vi "Normal Coefficient of Variation PDF SDV.vi"(8 "error in":errorcluster, 10 "n":i32=100, 11 "CV":dbl=0.21) -> (0 "error out":errorcluster={"status"=FALSE, "code"=-23026, "source"="Scale range exceeded"}, 1 "Baseline":dbl, 2 "SDV":dbl, 3 "Mean":dbl, 4 "Fit Result String":string="CV PDF  Gaussian LM Least Square Fit:\nAmplitude: 25.528592 ± 0.013986\nCenter: 0.210423 ± 9.838581E-6\nSDV: 0.015489 ± 9.825245E-6\nFWHM: 0.036473 ± 2.313668E-5\nIntegral: 991.140471\nMSE: 0.060195\nR^2: 0.999786\n")   [LabVIEW 2021, in "Math.lvlib"]
uses:
  Math.lvlib
  85f3da7c-8858-4d9f-a12c-d9901bcd4fde.vi
  Fits/Fits.lvlib
  <vilib>/Utility/miscctls.llb/LVPointDoubleTypeDef.ctl
  Fits/Fit Models.ctl
  Fits/Fit Plot Request Information.ctl
  Arrays/Linear Ramp End Options.ctl
  Arrays/Arrays.lvlib
  Fits/Nonlinear Fit Method.ctl
  Fits/Ramp Type.ctl
  Fits/Residual Type.ctl
  Fits/Non-linear Fitting Algorithm.ctl
  Fits/Fit Settings.ctl
  Fits/IRF(X)PSED/Fit Weights Type v2.ctl
panel:
  out "Fit Parameter Values":dbl[](array[numeric])
  out "XY Graph":cluster{"X Array":dbl[], "Y Array":dbl[]}[](graph)
  in  "# Steps (1)":i32=1000
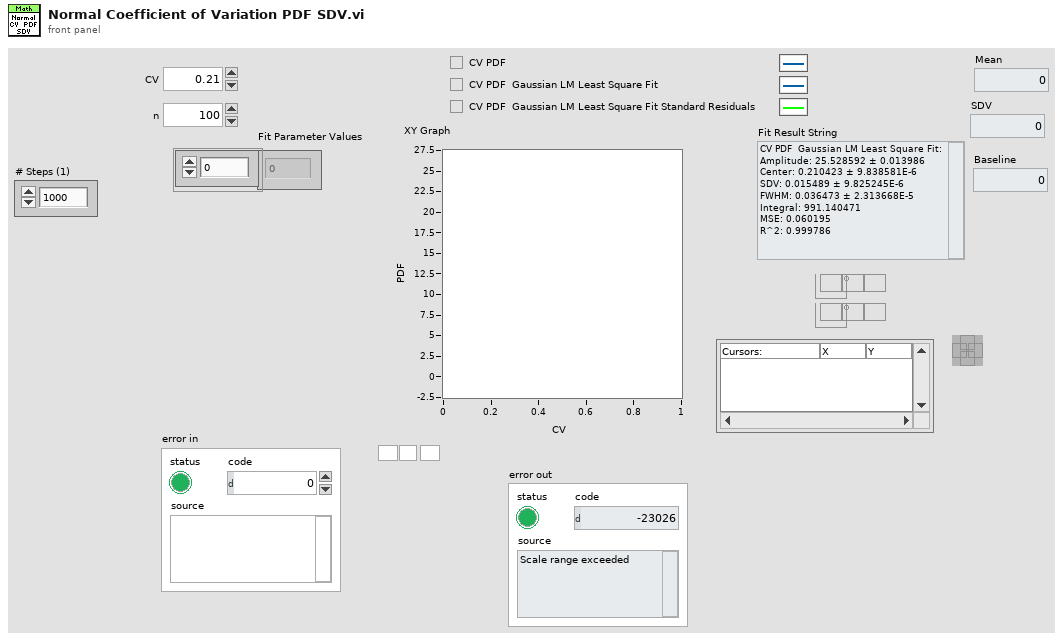
[diagram p1: front panel]
types:
  T1 = typedef "Fits.lvlib/Fit Settings.ctl" = cluster{"Use Original Plot # Points":bool, "# Fit Plot Points":u32, "Fitting Method":T2, "Weighted Fit":T3, "Show All Fit Components":bool, "Axis Type":T4, "Show Fit Residuals":bool, "Residual Type":T5, "Fitting Algorithm":T6, "Show Confidence Interval":bool, "Confidence Level":dbl}
  T2 = typedef "Fits.lvlib/Nonlinear Fit Method.ctl" = enum16{"Least Square", "Least Absolute Residual", "Bisquare", "MLE"}
  T3 = typedef "Fits.lvlib/Fit Weights Type v2.ctl" = enum16{"Unweighted", "1/Variance (Neyman)", "1/Variance (Pearson)", "Best of All"}
  T4 = typedef "Fits.lvlib/Ramp Type.ctl" = u16
  T5 = typedef "Fits.lvlib/Residual Type.ctl" = enum16{"Standard", "Normalized", "Reduced"}
  T6 = typedef "Fits.lvlib/Non-linear Fitting Algorithm.ctl" = enum16{"Levenberg-Marquardt", "Trust-Region Dogleg"}
  T7 = typedef "Arrays.lvlib/Linear Ramp End Options.ctl" = enum16{"Include Min/Exclude Max", "Exclude Min/Include Max", "Include Both Ends", "Exclude Both Ends"}
  T8 = typedef "LVPointDoubleTypeDef.ctl" = cluster{"X":dbl, "Y":dbl}
  T9 = typedef "Fits.lvlib/Fit Models.ctl" = enum16{"Select a Fit Model...", "           Single Peak", "Gaussian", "Asymmetric Gaussian", "Lorentzian", "Asymmetric Lorentzian", "Gaussian/Lorentzian", "Lorentzian/Gaussian", "           Double Peak", "Two Gaussians", "Two Asymmetric Gaussians", "Two H-Connected Gaussians", "Two T-Connected Gaussians", "Two H-Connected Asymmetric Gaussians", "Two T-Connected Asymmetric Gaussians", "           Triple Peak", "Three Gaussians", "Three Asymmetric Gaussians", "              Decays", "1-Exponential", "IRF*PSED", "2-Exponentials", "            Power Law", "Power Law", "Power Law with Offset", "               ACF", "2D Gaussian ACF", "2D Gaussian + Blinking ACF", "2D Gaussian + Flow ACF", "3D Gaussian ACF", "3D Gaussian + Blinking ACF", "             Multiplot", "2D Gaussian ACF & 2D Gaussian + Flow ACF"}
  T10 = typedef "Fits.lvlib/Fit Plot Request Information.ctl" = cluster{"XY Graph Ref":refnum<vi>, "Mouse Coordinates":T8, "Fit Model":T9, "Plot Index":i32}
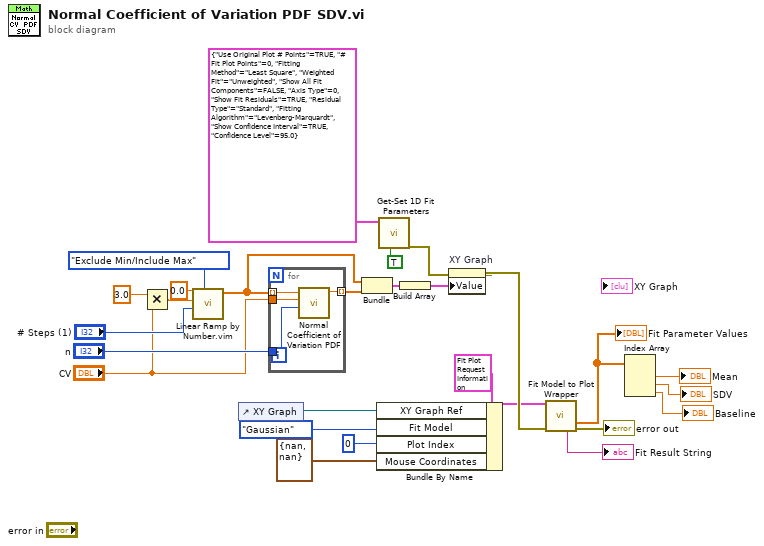
[diagram p0: block diagram]
diagram:
  n1 = Multiply(x=3.0, y="CV") -> (x*y=w9:dbl)
  n2 = call "Linear Ramp by Number.vim"("Options"=Linear_Ramp_End_Options."Exclude Min/Include Max", "# Steps (1)"="# Steps (1)", "End (1)"=w9, "Start (0)"=0.0 ("x")) -> ("Ramp"=w24:dbl[])  [unwired: 5 in, 2 out]
  n3 = control-ref of="XY Graph"() -> (w18:refnum<vi>)
  n4 = for {
    tunnel: w24 -> [w31] mode=indexing
    tunnel: "CV" -> [w30]
    tunnel: "n" -> [w29]
    tunnel: [w28] -> w25 mode=indexing
    n5 = call "Normal Coefficient of Variation PDF.vi"("n"=w29, "CV"=w30, "x"=w31) -> ("PDF (x)"=w28:dbl)  [unwired: 7 in, 1 out]
  }
  n6 = Bundle("Ramp"=w24, w25) -> (w23:cluster{"Ramp":dbl[], dbl[]})  [unwired: 1 in]
  n7 = Bundle By Name(cluster=T10 {"XY Graph Ref"=refnum, "Mouse Coordinates"={"X"=0.0, "Y"=0.0}, "Fit Model"=enum."Gaussian", "Plot Index"=0} ("Fit Plot Info"), "XY Graph Ref"=w18, "Fit Model"=Fit_Models."Gaussian", "Plot Index"=0, "Mouse Coordinates"=T8 {"X"=nan, "Y"=nan}) -> (w19:T10)
  n8 = call "Get-Set 1D Fit Parameters.vi"("Get(F)/Set"=TRUE, "Fit Settings"=T1 {"Use Original Plot # Points"=TRUE, "# Fit Plot Points"=0, "Fitting Method"=enum."Least Square", "Weighted Fit"=enum."Unweighted", "Show All Fit Components"=FALSE, "Axis Type"=0, "Show Fit Residuals"=TRUE, "Residual Type"=enum."Standard", "Fitting Algorithm"=enum."Levenberg-Marquardt", "Show Confidence Interval"=TRUE, "Confidence Level"=95.0}) -> ("Error Out"=w11:errorcluster)  [unwired: 6 in, 3 out]
  n9 = Build Array(w23) -> (w21:cluster{"Ramp":dbl[], dbl[]}[])
  n10 = property on="XY Graph" class="XYGraph (strict)"(error in=w11, "Value"=w21) -> (error out=w20:errorcluster)  [unwired: 1 in, 1 out]
  n11 = call "Fit Model to Plot Wrapper.vi"("Fit Plot Info"=w19, "error in (no error)"=w20) -> ("Fit Parameter Values"=w4:dbl[], "Fit Result String"=→"Fit Result String":string, "error out"=→"error out":errorcluster)  [unwired: 5 in, 6 out]
  "Fit Parameter Values" <- w4
  n12 = Index Array(array=w4) -> (element #1=→"Mean":dbl, element #2=→"SDV":dbl, element #3=→"Baseline":dbl)  [unwired: 3 in]
